vi "Main.vi"() -> ()   [LabVIEW 2015]
doc: "VI Main."
uses:
  UndoLibrary/Controls/cluster_Control Value.ctl
  UndoLibrary/UndoLibrary.lvlib
panel:
  in  "City":string
  in  "Sex":enum32{"Female", "Male"}(radio)
  in  "Birthday":timestamp format="%<%x>T"
  in  "Name":string
  in  "stop":bool
  # "Run-Time Menu uses \"Edit\" User item.\n\nThe code works both in Development mode and in exe."
  # "Actual application visible front panel"
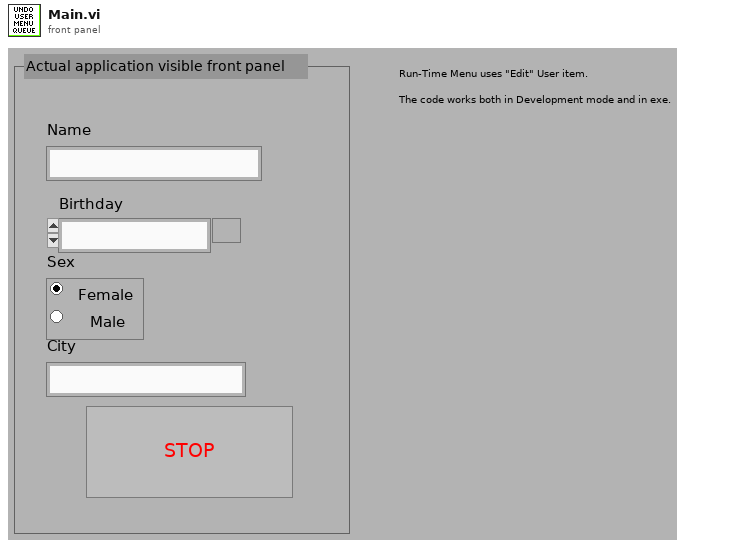
[diagram p1: front panel]
types:
  T1 = typedef "UndoLibrary.lvlib/cluster_Control Value.ctl" = cluster{"Index":i32, "Variant Data":variant}
  T2 = typedef "UndoLibrary.lvlib/cluster_All Queue.ctl" = cluster{"Current Queue":refnum<queue>, "Undo Queue":refnum<queue>, "Redo Queue":refnum<queue>}
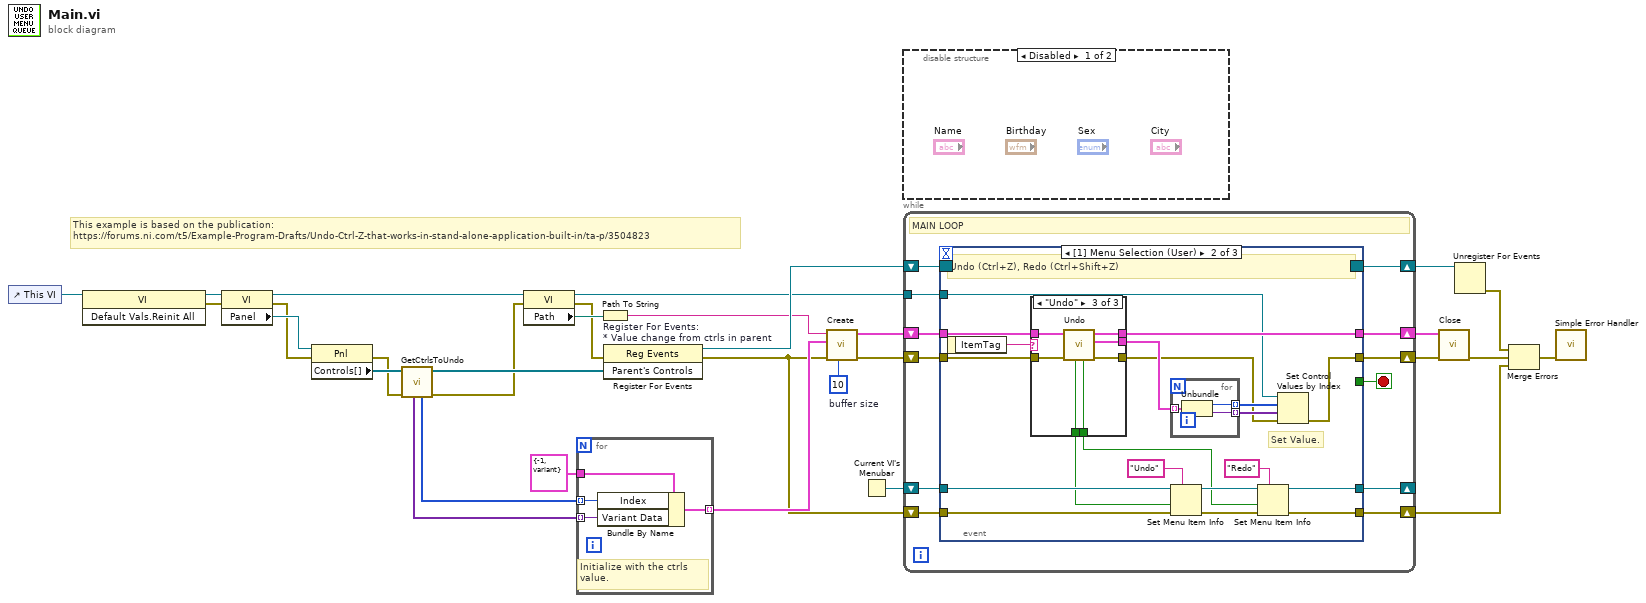
[diagram p0: block diagram]
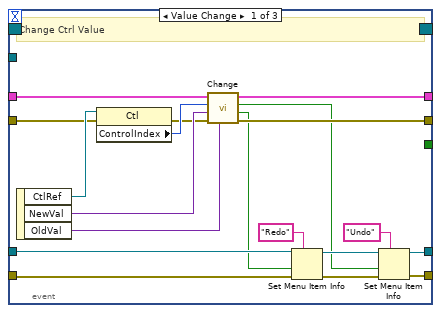
[diagram p3: hidden frame]
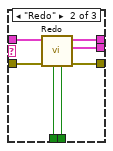
[diagram p5: hidden frame]
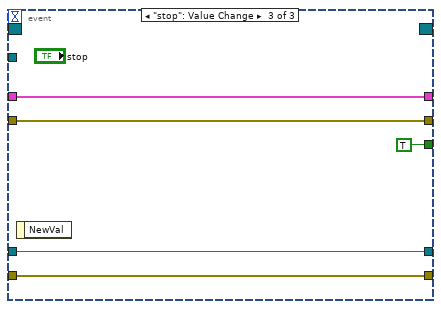
[diagram p6: hidden frame]
diagram:
  w28 = 10  # buffer size
  # "This example is based on the publication:\nhttps://forums.ni.com/t5/Example-Program-Drafts/Undo-Ctrl-Z-that-works-in-stand-alone-application-built-in/ta-p/3504823"
  n1 = control-ref of="This VI"() -> (w15:refnum<vi>)
  n2 = invoke class="VI" method="Default Vals.Reinit All"(reference=w15) -> (reference out=w14:refnum<vi>, error out=w13:errorcluster)  [unwired: 2 in, 1 out]
  n3 = property class="VI"(reference=w14, error in=w13) -> (reference out=w16:refnum<vi>, error out=w12:errorcluster, "Panel"=w31:refnum<vi>)
  n4 = property class="Pnl"(reference=w31, error in=w12) -> (error out=w10:errorcluster, "Controls[]"=w11:refnum<vi>[])  [unwired: 1 out]
  n5 = call "GetCtrlsToUndo.vi"("error in"=w10, "References\nfor Controls\non parent"=w11) -> ("error out"=w8:errorcluster, "Parent's Controls"=w9:refnum<vi>[], "Index"=w7:i32[], "Initial Values"=w6:variant[])  [unwired: 6 in]
  n6 = property class="VI"(reference=w16, error in=w8) -> (reference out=w20:refnum<vi>, error out=w17:errorcluster, "Path"=w19:path)
  n7 = for {
    tunnel: [w35] -> w29 mode=indexing
    tunnel: w7 -> [w34] mode=indexing
    tunnel: w6 -> [w33] mode=indexing
    tunnel: T1 {"Index"=-1, "Variant Data"=variant} ("Control Value") -> [w32]
    # "Initialize with the ctrls\nvalue."
    n8 = Bundle By Name(cluster=w32, "Index"=w34, "Variant Data"=w33) -> (w35:T1)
  }
  n9 = Path To String(path=w19) -> (string=w18:string)
  n10 = register-events "Register For Events:\n* Value change from ctrls in parent"(error in=w17, w9) -> (reference out=w23:refnum<event-registration>, error out=w2:errorcluster)  [unwired: 1 in]
  n11 = call "Create.vi"("buffer size (10)"=w28, "error in (no error)"=w2, "Ctrl Val.Set All"=w29, "name (unnamed)"=w18) -> ("error out"=w27:errorcluster, "All Queue out"=w30:T2)  [unwired: 6 in]
  n12 = Current VI's Menubar() -> (w3:refnum<k9>)
  n13 = disable-structure shown="Disabled" {
    frame Disabled {
    }
    frame Enabled {
    }
  }
  n14 = while {
    shift-right: [w44] -> w26
    shift-left: w30 -> [w46]
    shift-right: [w43] -> w25
    shift-left: w27 -> [w45]
    tunnel: w20 -> [w42]
    shift-right: [w40] -> w22
    shift-left: w23 -> [w41]
    shift-right: [w37] -> _
    shift-left: w3 -> [w39]
    shift-right: [w36] -> w1
    shift-left: w2 -> [w38]
    stop <- w47 stop-if-true
    # "MAIN LOOP"
    n15 = event shown="[1] Menu Selection (User)" {
      selector: w41 -> [_ _ _]
      dyn-events: [_ _ _] -> w40
      timeout: _ -> [_ _ _]
      tunnel: [w65 w82 w109] -> w44
      tunnel: w46 -> [w66 w83 w109]
      tunnel: [_ _ TRUE] -> w47
      tunnel: w45 -> [w59 w81 w108]
      tunnel: [w61 w78 w108] -> w43
      tunnel: w42 -> [_ w80 _]
      tunnel: w39 -> [w51 w72 w107]
      tunnel: w38 -> [w50 w71 w106]
      tunnel: [w53 w70 w107] -> w37
      tunnel: [w52 w69 w106] -> w36
      event Value Change {
        # "Change Ctrl Value"
        n16 = event-data() -> ("CtlRef"=w63:refnum<vi>, "NewVal"=w60:variant, "OldVal"=w64:variant)  [unwired: 1 in]
        n17 = property class="Ctl"(reference=w63, error in=w59) -> (error out=w58:errorcluster, "ControlIndex"=w62:i32)  [unwired: 1 out]
        n18 = call "Change.vi"("OldVal"=w64, "error in (no error)"=w58, "NewVal"=w60, "Control Index"=w62, "All Queue in"=w66) -> ("error out"=w61:errorcluster, "Redo Enable"=w48:bool, "Undo Enable"=w49:bool, "All Queue out"=w65:T2)  [unwired: 3 in]
        n19 = Set Menu Item Info(7:"Redo" ("item tag"), 8:w50, 9:w48, 11:w51) -> (0:w56:errorcluster, 3:w57:refnum<k9>)  [unwired: 3 out]
        n20 = Set Menu Item Info(7:"Undo" ("item tag"), 8:w56, 9:w49, 11:w57) -> (0:w52:errorcluster, 3:w53:refnum<k9>)  [unwired: 3 out]
      }
      event Menu Selection (User) {
        # "Set Value."
        # "Undo (Ctrl+Z), Redo (Ctrl+Shift+Z)"
        n21 = event-data() -> ("ItemTag"=w77:string)  [unwired: 1 in]
        n22 = case shown="\"Undo\"" w77 {
          tunnel: [_ w92 w102] -> w86
          tunnel: w83 -> [w88 w95 w101]
          tunnel: [w88 w93 w100] -> w82
          tunnel: w81 -> [w87 w94 w99]
          tunnel: [w87 w91 w98] -> w79
          tunnel: [_ w90 w97] -> w68
          tunnel: [_ w89 w96] -> w67
          frame Default {
          }
          frame "Redo" {
            n23 = call "Redo.vi"("error in (no error)"=w94, "All Queue in"=w95) -> ("error out"=w91:errorcluster, "Ctrl Val.Get All"=w92:T1[], "All Queue out"=w93:T2, "Redo Enable"=w89:bool, "Undo Enable"=w90:bool)  [unwired: 5 in]
          }
          frame "Undo" {
            n24 = call "Undo.vi"("error in (no error)"=w99, "All Queue in"=w101) -> ("error out"=w98:errorcluster, "Ctrl Val.Get All"=w102:T1[], "All Queue out"=w100:T2, "Redo Enable"=w96:bool, "Undo Enable"=w97:bool)  [unwired: 5 in]
          }
        }
        n25 = for {
          tunnel: w86 -> [w105] mode=indexing
          tunnel: [w104] -> w85 mode=indexing
          tunnel: [w103] -> w84 mode=indexing
          n26 = Unbundle(w105) -> ("Index"=w104:i32, "Variant Data"=w103:variant)
        }
        n27 = Set Menu Item Info(7:"Undo" ("item tag"), 8:w71, 9:w68, 11:w72) -> (0:w75:errorcluster, 3:w76:refnum<k9>)  [unwired: 3 out]
        n28 = Set Menu Item Info(7:"Redo" ("item tag"), 8:w75, 9:w67, 11:w76) -> (0:w69:errorcluster, 3:w70:refnum<k9>)  [unwired: 3 out]
        n29 = Set Control Values by Index(0:w80, 1:w85, 2:w84, 3:w79) -> (11:w78:errorcluster)
      }
      event "stop": Value Change {
        n30 = event-data() -> ()  [unwired: 1 in, 1 out]
      }
    }
  }
  n31 = call "Close.vi"("error in (no error)"=w25, "All Queue in"=w26) -> ("error out"=w24:errorcluster)  [unwired: 9 in]
  n32 = Unregister For Events(event registration refnum=w22) -> (error out=w21:errorcluster)  [unwired: 1 in]
  n33 = Merge Errors(w21, w24, w1) -> (w5:errorcluster)
  n34 = call <vilib>:"Simple Error Handler.vi"("error in (no error)"=w5) -> ()  [unwired: 4 in, 5 out]
